vi "Application_Init.vi"(8 "ErrorIn":errorcluster, 11 "ReferenceIn":refnum<class "Application.lvclass"> caption="This control should only be used when\na sub class is inheriting this class") -> (0 "ErrorOut":errorcluster, 3 "ReferenceOut":refnum<class "Application.lvclass"> caption="This indicator should only be used when\na sub class is inheriting this class")   [LabVIEW 2021, in "Application.lvclass"]
uses:
  Application.lvclass
  05b08f85-94a6-4d81-b7cc-f03ecc06fb25.vi
  <vilib>/TriekselSoft/TracerLibrary/TracerLibrary/Tracer/protected/SendMessage.vi
  <vilib>/TriekselSoft/TracerLibrary/TracerLibrary/Tracer/protected/Timestamp.vi
  05b08f85-94a6-4d81-b7cc-f03ecc06fb25.vi/f75db090-0877-4668-94fb-75c2140b1617.vi
  <vilib>/TriekselSoft/TracerLibrary/TracerLibrary/Tracer/Tracer_Level-Debug.vi
  <vilib>/JDP Science/JSONtext/Variant to JSON Text.vi
  <vilib>/TriekselSoft/TracerLibrary/TracerLibrary/Tracer/protected/Tracer_ClassAttributes.vi
  <vilib>/JDP Science/JSONtext/LVClass Serializer/JSONtext LVClass Serializer.lvclass
  Application.lvclass/Application.ctl
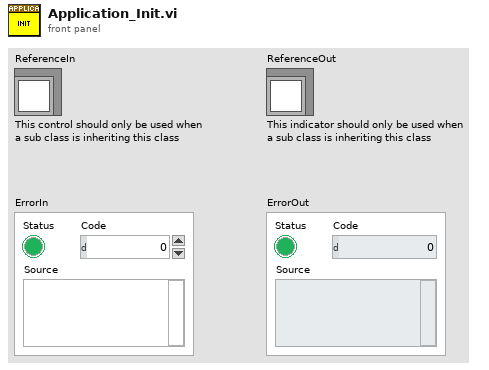
[diagram p1: front panel]
types:
  T1 = typedef "Application.lvclass/ObjectAttributes.ctl" = cluster{"Objects":variant, "BasePath":path, "Application":refnum<class "Application.lvclass">}
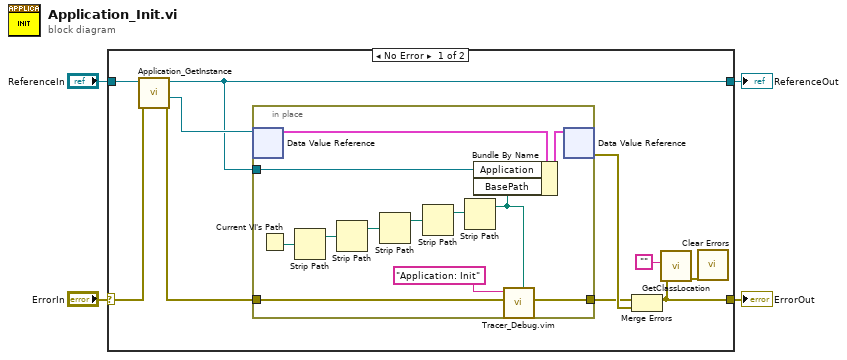
[diagram p0: block diagram]
diagram:
  n1 = case shown="No Error" "ErrorIn" {
    selector: "ErrorIn" -> [w13 w28]
    tunnel: [w10 w28] -> w3
    tunnel: "ReferenceIn" -> [w8 w27]
    tunnel: [w6 w27] -> w1
    frame No Error {
      n2 = call "Application_GetInstance.vi"("ErrorIn"=w13, "ReferenceIn"=w8) -> ("ErrorOut"=w12:errorcluster, "DVRRefOut"=w7:refnum<data-value>, "ReferenceOut"=w6:refnum<class "Application.lvclass">)  [unwired: 5 in, 2 out]
      n3 = in-place {
        in-place-border: w12 -> [w26]
        in-place-border: [w25] -> w11
        in-place-border: w6 -> [w19]
        n4 = in-place-dvr #1(w7) -> (w23:T1)  [unwired: 1 out]
        n5 = Current VI's Path() -> (path=w22:path)
        n6 = Strip Path(path=w22) -> (stripped path=w21:path)  [unwired: 1 out]
        n7 = Strip Path(path=w21) -> (stripped path=w20:path)  [unwired: 1 out]
        n8 = Strip Path(path=w20) -> (stripped path=w18:path)  [unwired: 1 out]
        n9 = Strip Path(path=w18) -> (stripped path=w17:path)  [unwired: 1 out]
        n10 = Strip Path(path=w17) -> (stripped path=w15:path)  [unwired: 1 out]
        n11 = Bundle By Name(cluster=w23, "Application"=w19, "BasePath"=w15) -> (w24:T1)
        n12 = call "Tracer_Debug.vim"("Data"=w15, "error in (no error)"=w26, "Text"="Application: Init") -> ("error out"=w25:errorcluster)  [unwired: 8 in]
        n13 = in-place-dvr #1(w24) -> (w14:errorcluster)  [unwired: 1 out]
      }
      n14 = Merge Errors(w11, w14) -> (w10:errorcluster)
      n15 = call "GetClassLocation.vi"("Error In"=w10, "ClassString"="") -> ("Error Out"=w9:errorcluster)  [unwired: 8 in, 1 out]
      n16 = call <vilib>:"Clear Errors.vi"("error in (no error)"=w9) -> ()  [unwired: 5 in, 2 out]
    }
    frame Error {
    }
  }
  "ErrorOut" <- w3
  "ReferenceOut" <- w1
